vi "Wait for Pending Operation.vi"(8 "error in (no error)":errorcluster, 11 "VISA resource name":refnum<visa-resource-name>) -> (0 "error out":errorcluster, 3 "VISA resource name out":refnum<visa-resource-name>)   [LabVIEW 2018, in "LTB-1.lvlib" / "3150.lvlib"]
doc: "This VI prevents the device from executing any further commands or queries until the no-operation-pending flag becomes TRUE."
uses:
  3150.lvlib
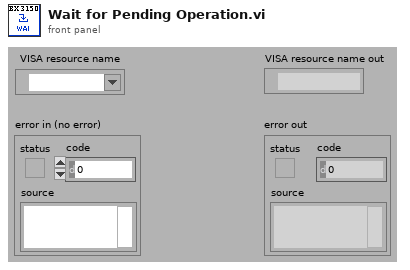
[diagram p1: front panel]
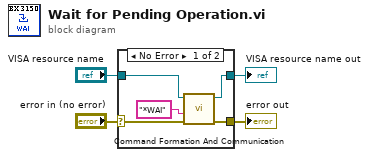
[diagram p0: block diagram]
diagram:
  n1 = case shown="No Error" "error in (no error)" {
    selector: "error in (no error)" -> [w9 w11]
    tunnel: [w8 w11] -> w1
    tunnel: [w7 w10] -> w3
    tunnel: "VISA resource name" -> [w5 w10]
    frame No Error {
      n2 = call "Command Formation And Communication.vi"("error in (no error)"=w9, "Command"="*WAI", "VISA resource name"=w5) -> ("error out"=w8:errorcluster, "VISA resource name out"=w7:refnum<visa-resource-name>)  [unwired: 1 in, 6 out]
    }
    frame Error {
    }
  }
  "VISA resource name out" <- w3
  "error out" <- w1
